vi "Load Configuration.vi"(6 "wait for reply (T)":bool=TRUE, 8 "error in":errorcluster, 10 "Setup":T1) -> (0 "error out":errorcluster, 1 "timed out?":bool)   [LabVIEW 2024, in "EtherCAT Model.lvlib"]
doc: "This loads the EtherCAT configuration.\n_____\nCreated using DQMH Event Scripter 7.0.1.1316."
uses:
  EtherCAT Model.lvlib
  EtherCAT Configuration.ctl
  Load Configuration Argument--cluster.ctl
  Load Configuration (Reply Payload)--cluster.ctl
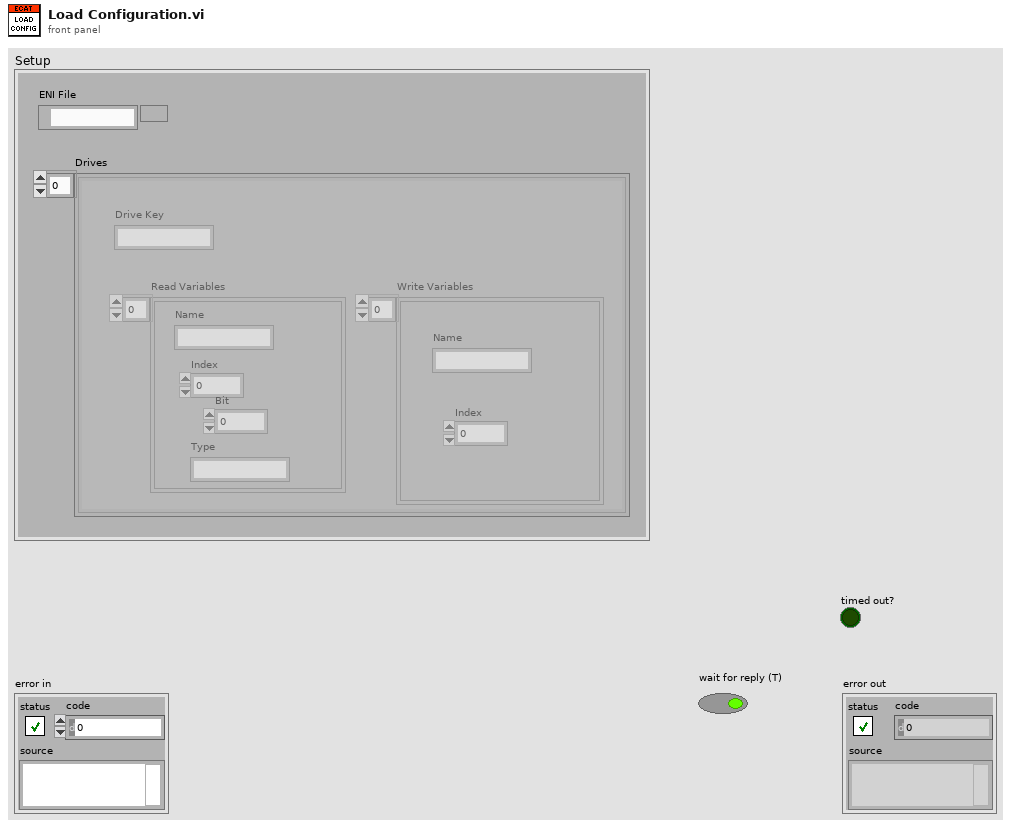
[diagram p1: front panel]
types:
  T1 = typedef "EtherCAT Configuration.ctl" = cluster{"ENI File":path, "Drives":cluster{"Drive Key":string, "Read Variables":cluster{"Name":string, "Index":u16, "Bit":u8, "Type":string}[], "Write Variables":cluster{"Name":string, "Index":u16}[]}[]}
  T2 = typedef "EtherCAT Model.lvlib/Load Configuration Argument--cluster.ctl" = cluster{"Setup":T1, "Wait Notifier":refnum<notifier>, "wait for reply":bool}
  T3 = typedef "EtherCAT Model.lvlib/Request Events--cluster.ctl" = cluster{"Stop Module":refnum<user-event>, "Show Panel":refnum<user-event>, "Hide Panel":refnum<user-event>, "Get Module Execution Status":refnum<user-event>, "Show Diagram":refnum<user-event>, "Load Configuration":refnum<user-event>}
  T4 = typedef "EtherCAT Model.lvlib/Load Configuration (Reply Payload)--cluster.ctl" = cluster{"error":errorcluster}
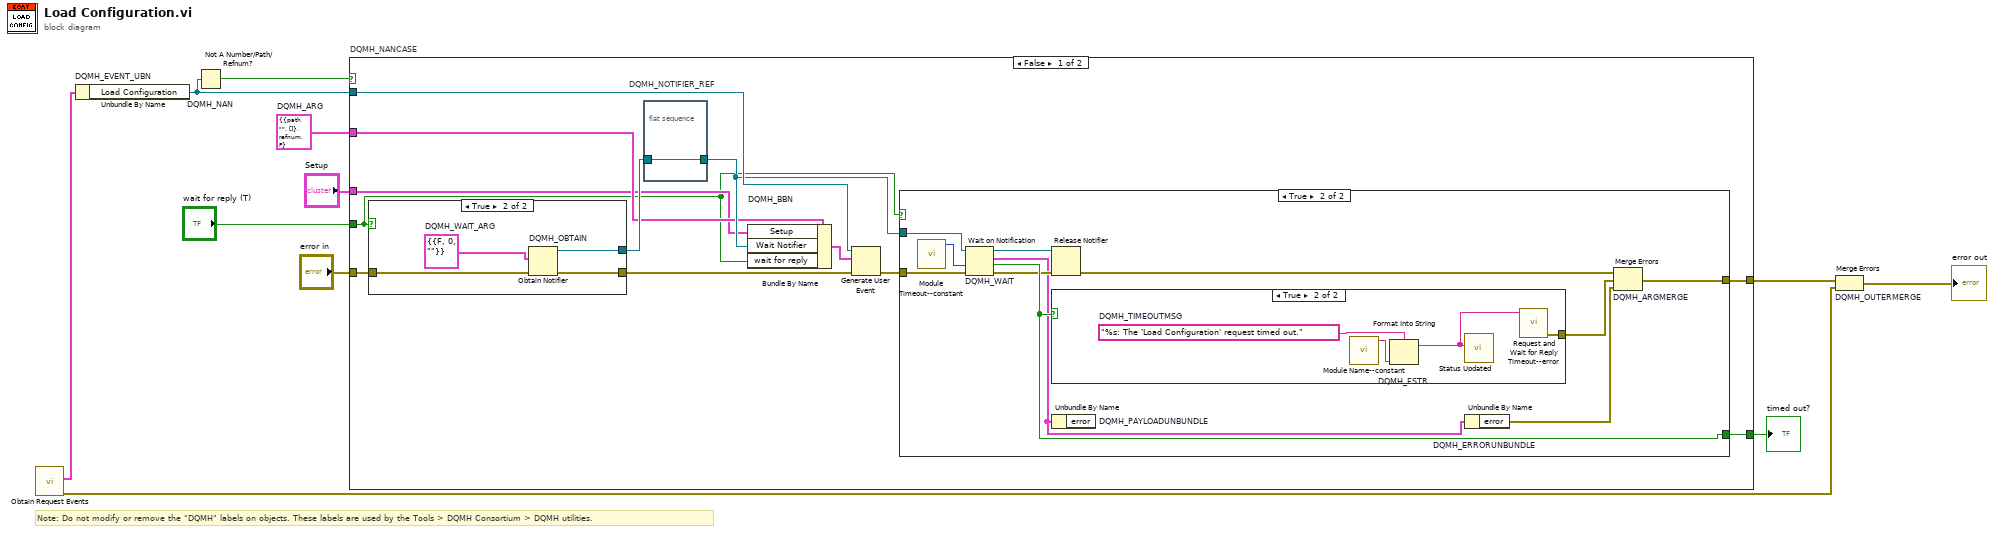
[diagram p0: block diagram]
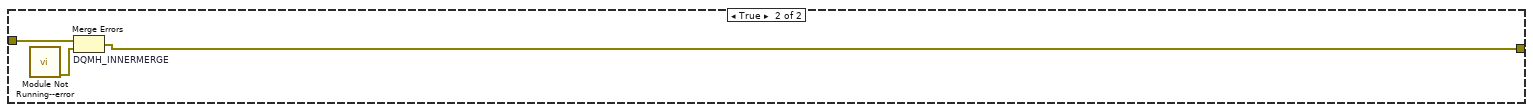
[diagram p5: hidden frame]
diagram:
  w5 = T2 {"Setup"={"ENI File"=path "", "Drives"=[]}, "Wait Notifier"=refnum, "wait for reply"=FALSE}  # DQMH_ARG
  # "Note: Do not modify or remove the \"DQMH\" labels on objects. These labels are used by the Tools > DQMH Consortium > DQMH utilities."
  n1 = call "Obtain Request Events.vi"() -> ("error out"=w2:errorcluster, "EtherCAT Model Request Events"=w1:T3)  [unwired: 10 in]
  n2 = Unbundle By Name "DQMH_EVENT_UBN"(w1) -> ("Load Configuration"=w9:refnum<user-event>)
  n3 = Not A Number/Path/Refnum? "DQMH_NAN"(number/path/refnum=w9) -> (NaN/Path/Refnum?=w8:bool)
  n4 = case "DQMH_NANCASE" shown="False" w8 {
    tunnel: "error in" -> [w23 w48]
    tunnel: w9 -> [w21 _]
    tunnel: [w18 w47] -> w6
    tunnel: [w19 _] -> w7
    tunnel: w5 -> [w14 _]
    tunnel: "Setup" -> [w13 _]
    tunnel: "wait for reply (T)" -> [w12 _]
    frame False {
      n5 = case shown="True" w12 {
        tunnel: w23 -> [w41 w45]
        tunnel: [w41 w44] -> w20
        tunnel: [_ w42] -> w16
        frame False {
        }
        frame True {
          w43 = T4 {"error"={"status"=FALSE, "code"=0, "source"=""}}  # DQMH_WAIT_ARG
          n6 = Obtain Notifier "DQMH_OBTAIN"(notification data type=w43, error in (no error)=w45) -> (notifier out=w42:refnum<notifier>, error out=w44:errorcluster)  [unwired: 2 in, 1 out]
        }
      }
      n7 = flat-sequence "DQMH_NOTIFIER_REF" {
        tunnel: w16 -> [w24]
        tunnel: [w24] -> w15
        frame #0 {
        }
      }
      n8 = Bundle By Name "DQMH_BBN"(cluster=w14, "Setup"=w13, "Wait Notifier"=w15, "wait for reply"=w12) -> (w17:T2)
      n9 = Generate User Event(user event=w21, event data cluster=w17, error in=w20) -> (error out=w22:errorcluster)  [unwired: 1 in, 1 out]
      n10 = case shown="True" w12 {
        tunnel: w22 -> [w25 w36]
        tunnel: w15 -> [_ w35]
        tunnel: [_ w33] -> w19
        tunnel: [w25 w32] -> w18
        frame False {
        }
        frame True {
          n11 = call "Module Timeout--constant.vi"() -> ("Module Timeout"=w26:i32)  [unwired: 11 in]
          n12 = Wait on Notification "DQMH_WAIT"(notifier=w35, timeout in ms (-1)=w26, error in (no error)=w36) -> (notifier out=w34:refnum<notifier>, notification=w27:T4, timed out?=w33:bool, error out=w31:errorcluster)  [unwired: 1 in]
          n13 = Release Notifier(notifier=w34, error in (no error)=w31) -> (error out=w30:errorcluster)  [unwired: 1 in, 2 out]
          n14 = case shown="True" w33 {
            tunnel: [_ w38] -> w28
            frame False {
            }
            frame True {
              w40 = "%s: The 'Load Configuration' request timed out."  # DQMH_TIMEOUTMSG
              n15 = call "Module Name--constant.vi"() -> ("Module Name"=w37:string)  [unwired: 11 in]
              n16 = Format Into String "DQMH_FSTR"(format string=w40, w37) -> (resulting string=w39:string)  [unwired: 2 in, 1 out]
              n17 = call "Status Updated.vi"("Status"=w39) -> ()  [unwired: 10 in, 1 out]
              n18 = call "Request and Wait for Reply Timeout--error.vi"("Error Message"=w39) -> ("error out"=w38:errorcluster)  [unwired: 10 in]
            }
          }
          n19 = Unbundle By Name "DQMH_PAYLOADUNBUNDLE"(w27) -> ()  [unwired: 1 out]
          n20 = Unbundle By Name "DQMH_ERRORUNBUNDLE"(w27) -> ("error"=w29:errorcluster)
          n21 = Merge Errors "DQMH_ARGMERGE"(w30, w28, w29) -> (w32:errorcluster)
        }
      }
    }
    frame True {
      n22 = call "Module Not Running--error.vi"() -> ("error out"=w46:errorcluster)  [unwired: 11 in]
      n23 = Merge Errors "DQMH_INNERMERGE"(w48, w46) -> (w47:errorcluster)
    }
  }
  "timed out?" <- w7
  n24 = Merge Errors "DQMH_OUTERMERGE"(w6, w2) -> (→"error out":errorcluster)
